vi "DataChunkingLabview.vi"() -> ()   [LabVIEW 2019]
uses:
  <vilib>/addons/database/NI_Database_API.lvlib
  MIs softarwer2/JSW BELLERA CODE/New gary MIS/Gary Coating Code MIS/Sub VIs/Thickness.llb/Thickness Global.vi
  <vilib>/addons/database/Connection.llb/DB Tools Open Connec (String).vi
  <vilib>/addons/database/Auxilliary.llb/DB Tools Parameter Dir.ctl
  <vilib>/addons/database/Auxilliary.llb/DB Tools DataTypes.ctl
  <vilib>/addons/database/Auxilliary.llb/DB Tools Parameter Info.ctl
  <vilib>/addons/database/Command.llb/Cmd Set Parameter Value (C).vi
  <vilib>/addons/database/Auxilliary.llb/DB Tools Format Datetime String (Time Stamp).vi
  <vilib>/addons/database/Command.llb/Cmd Execute.vi
  <vilib>/addons/database/Recordset.llb/Rec Fetch Recordset Data (CR).vi
  <vilib>/addons/database/Command.llb/Cmd Delete.vi
  <vilib>/addons/database/Recordset.llb/Rec Destroy - Command.vi
panel:
  out "size(s)":i32[](array[numeric])
  in  "offset for Data":dbl
  in  "?":dbl
  out "no of iteration":i32
  out "Array":variant[][][](array[variant])
  in  "From  Date":timestamp
  out "Tota records":variant[][](array[variant])
  out "no of records from db":i32
  in  "To Date":timestamp
  out "element":variant
  out "initialized array":variant[](array[variant])
  out "date string 3":string
  out "time string 2":string
  out "date string 4":string
  out "time string 3":string
types:
  T1 = typedef "NI_Database_API.lvlib/Conn ObjectReference.ctl" = refnum<k1>
  T2 = typedef "NI_Database_API.lvlib/DB Tools Parameter Info.ctl" = cluster{"parameter name":string, "type":T3, "direction":T4, "value":variant}
  T3 = typedef "NI_Database_API.lvlib/DB Tools DataTypes.ctl" = enum16{"String", "Long (I32)", "Single (SGL)", "Double (DBL)", "Date/Time", "Binary"}
  T4 = typedef "NI_Database_API.lvlib/DB Tools Parameter Dir.ctl" = enum32{"Input", "Output", "Input/Output", "Return Value"}
  T5 = typedef "NI_Database_API.lvlib/Cmd ObjectReference.ctl" = refnum<k1>
  T6 = typedef "NI_Database_API.lvlib/Cmd-Rec Object Reference.ctl" = refnum<k1>
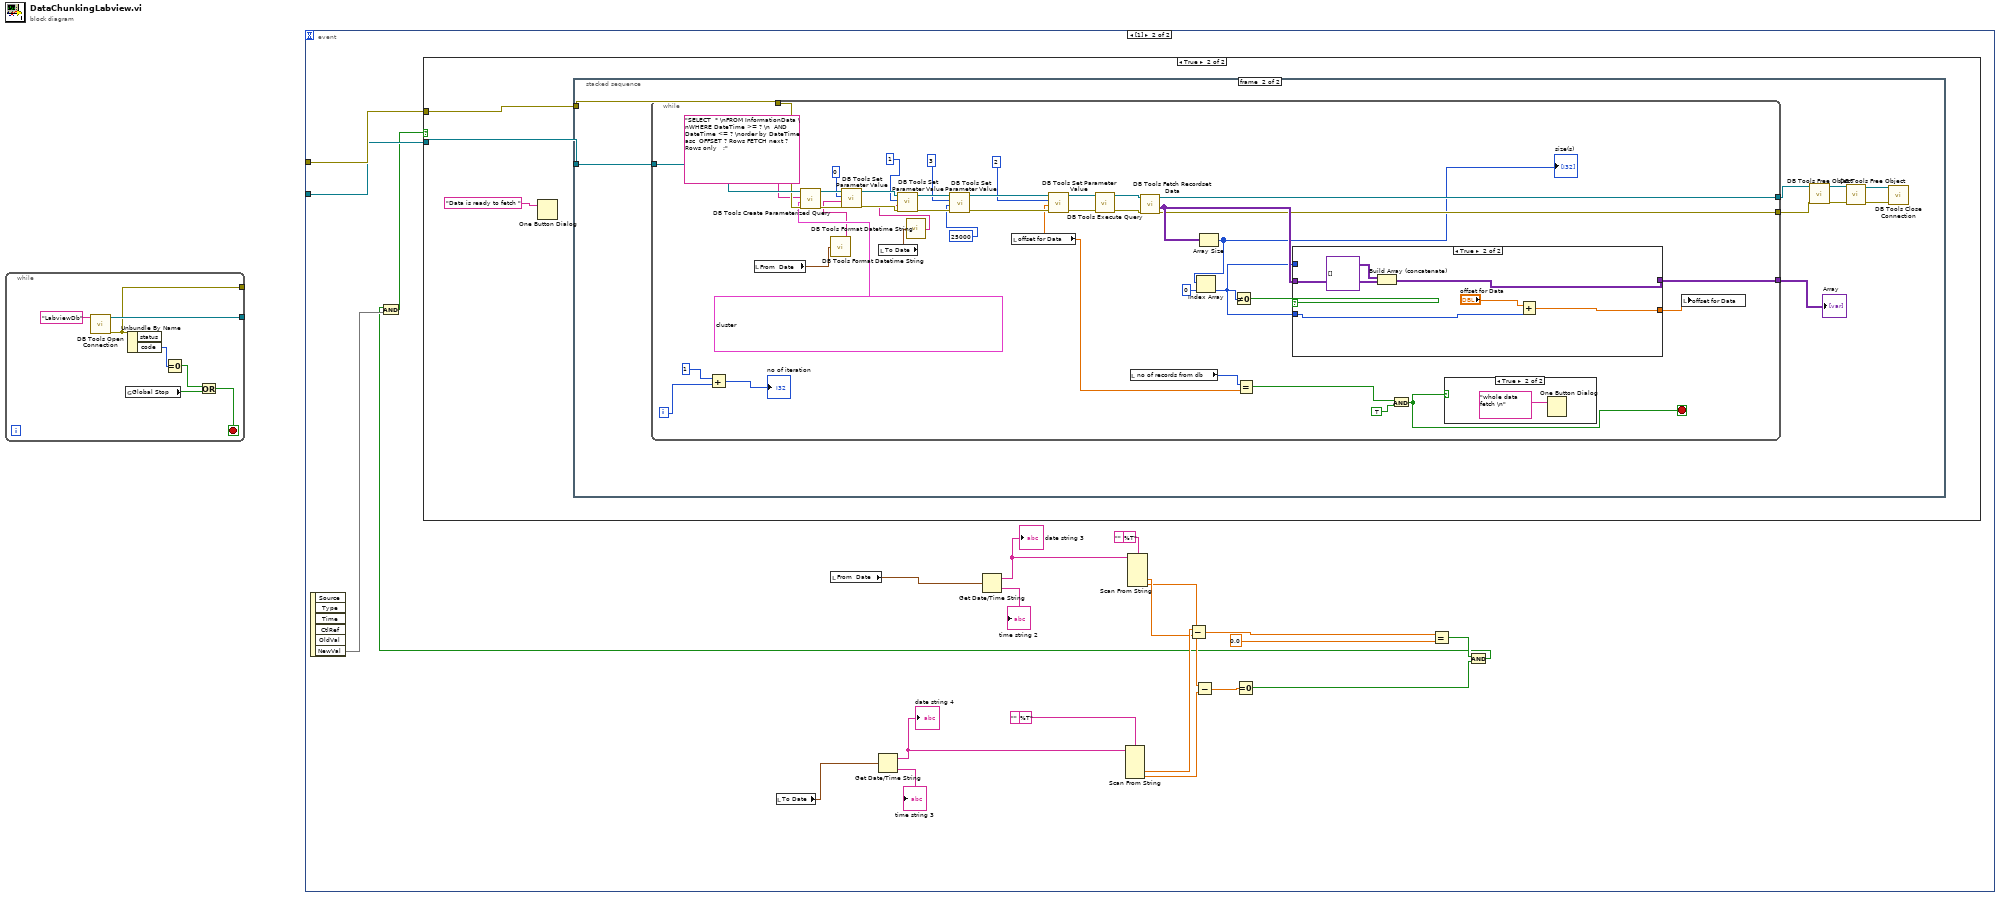
[diagram p0: block diagram]
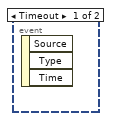
[diagram p2: hidden frame]
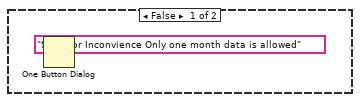
[diagram p3: hidden frame]
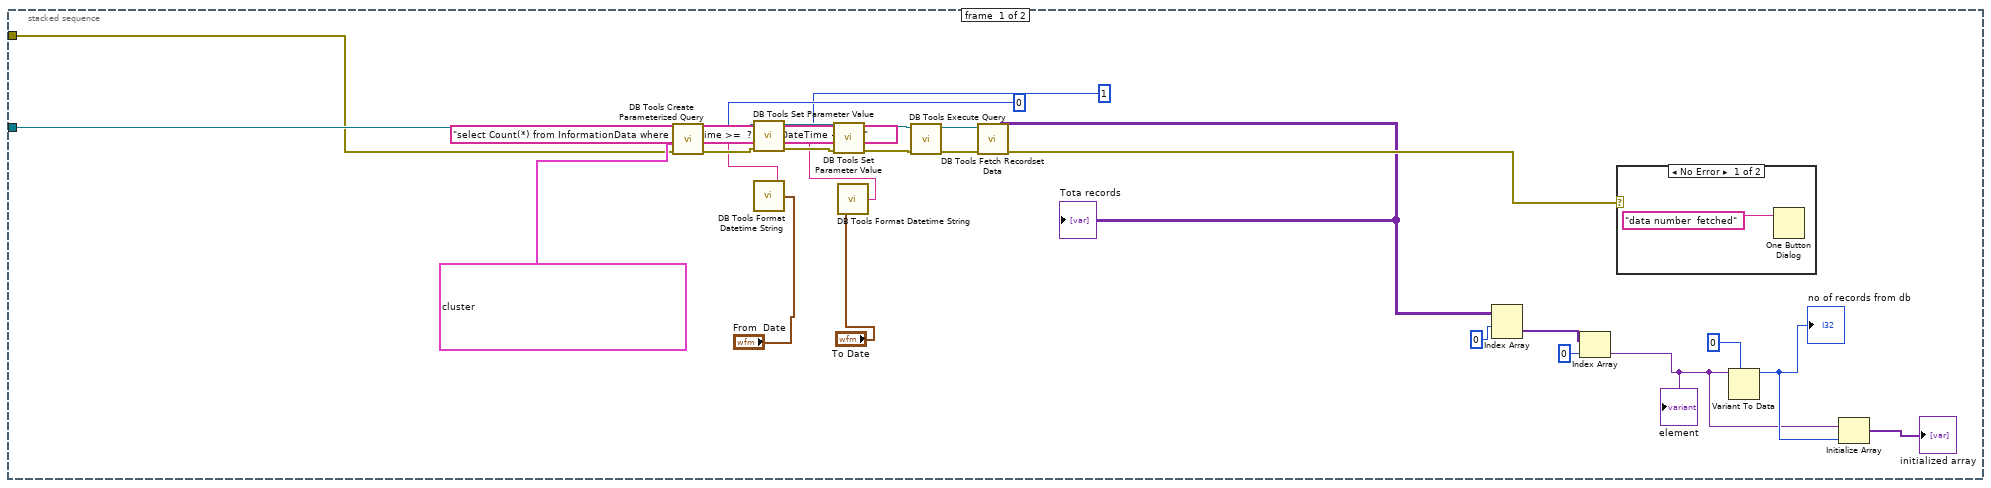
[diagram p4: hidden frame]
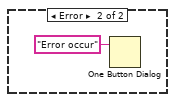
[diagram p5: hidden frame]
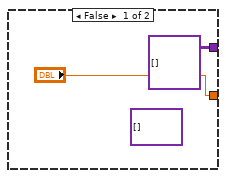
[diagram p7: hidden frame]
diagram:
  n1 = while {
    tunnel: [w2] -> _
    tunnel: [w1] -> _
    stop <- w3 stop-if-true
    n2 = call-poly <vilib>:"DB Tools Open Connection.vi"("connection information"="LabviewDb") -> ("error out"=w1:errorcluster, "connection reference"=w2:T1)  [unwired: 7 in]
    n3 = global read "Thickness Global.vi" "Global Stop"() -> (w4:bool)
    n4 = Unbundle By Name(w1) -> ("code"=w6:i32)  [unwired: 1 out]
    n5 = Equal To 0?(x=w6) -> (x = 0?=w5:bool)
    n6 = Or(x=w5, y=w4) -> (x .or. y?=w3:bool)
  }
  n7 = event shown="[1]" {
    selector: _ -> [_ _]
    dyn-events: _ -> [_ _]
    timeout: _ -> [_ _]
    tunnel: _ -> [_ w29]
    tunnel: _ -> [_ w28]
    event Timeout {
      n8 = event-data() -> ()  [unwired: 1 in, 3 out]
    }
    event #1 (no event record) {
      (unwired) "%T" ("format string")
      (unwired) "%T" ("format string")
      n9 = event-data() -> ("NewVal"=w27)  [unwired: 1 in, 5 out]
      n10 = local read "To Date"() -> (w8:timestamp)
      n11 = local read "From  Date"() -> (w9:timestamp)
      n12 = Get Date/Time String(seconds (now)=w8) -> (date string=w21:string, time string=→"time string 3":string)  [unwired: 2 in]
      "date string 4" <- w21
      n13 = Get Date/Time String(seconds (now)=w9) -> (date string=w24:string, time string=→"time string 2":string)  [unwired: 2 in]
      "date string 3" <- w24
      n14 = Scan From String(format string="", input string=w21) -> (output 2=w19:dbl, output 3=w14:dbl)  [unwired: 6 in, 3 out]
      n15 = Scan From String(format string="", input string=w24) -> (output 2=w18:dbl, output 3=w15:dbl)  [unwired: 6 in, 3 out]
      n16 = Subtract(x=w19, y=w18) -> (x-y=w16:dbl)
      n17 = Subtract(x=w15, y=w14) -> (x-y=w13:dbl)
      n18 = Equal To 0?(x=w13) -> (x = 0?=w11:bool)
      n19 = Equal?(x=w16, y=0.0) -> (x = y?=w12:bool)
      n20 = And(x=w12, y=w11) -> (x .and. y?=w10:bool)
      n21 = And(x=w10, y=w27) -> (x .and. y?=w26:bool)
      n22 = case shown="True" w26 {
        tunnel: w29 -> [_ w31]
        tunnel: w28 -> [_ w32]
        frame False {
          n23 = One Button Dialog(message="Sorry for Inconvience Only one month data is allowed") -> ()  [unwired: 1 in, 1 out]
        }
        frame True {
          n24 = One Button Dialog(message="Data is ready to fetch ") -> ()  [unwired: 1 in, 1 out]
          n25 = stacked-sequence {
            tunnel: w32 -> [w45 w71]
            tunnel: w31 -> [w44 w70]
            frame #0 {
              n26 = call <vilib>:"DB Tools Create Parameterized Query.vi"("error in (no error)"=w44, "parameters"=T2[] [{"parameter name"="fromDate", "type"=enum."Date/Time", "direction"=enum."Input", "value"=variant}, {"parameter name"="toDate", "type"=enum."Date/Time", "direction"=enum."Input", "value"=variant}], "SQL query"="select Count(*) from InformationData where  DateTime >=  ?  AND DateTime <= ?;  ", "connection reference"=w45) -> ("error out"=w57:errorcluster, "command reference"=w58:T5)  [unwired: 3 in, 1 out]
              n27 = call-poly <vilib>:"DB Tools Format Datetime String.vi"("time stamp"="From  Date") -> ("date/time string"=w55:string)
              n28 = call-poly <vilib>:"DB Tools Set Parameter Value.vi"("error in (no error)"=w57, "value"=w55, "parameter index"=0, "command reference"=w58) -> ("error out"=w53:errorcluster, "command reference out"=w54:T5)  [unwired: 4 in]
              n29 = call-poly <vilib>:"DB Tools Format Datetime String.vi"("time stamp"="To Date") -> ("date/time string"=w41:string)
              n30 = call-poly <vilib>:"DB Tools Set Parameter Value.vi"("error in (no error)"=w53, "value"=w41, "parameter index"=1, "command reference"=w54) -> ("error out"=w50:errorcluster, "command reference out"=w51:T5)  [unwired: 4 in]
              n31 = call-poly <vilib>:"DB Tools Execute Query.vi"("error in (no error)"=w50, "command reference"=w51) -> ("error out"=w48:errorcluster, "command-recordset reference"=w49:T6)  [unwired: 6 in]
              n32 = call-poly <vilib>:"DB Tools Fetch Recordset Data.vi"("error in (no error)"=w48, "command-recordset reference"=w49) -> ("error out"=w47:errorcluster, "recordset data"=w40:variant[][])  [unwired: 3 in, 1 out]
              "Tota records" <- w40
              n33 = Index Array(array=w40, index (row)=0 ("index")) -> (element=w39:variant[])  [unwired: 1 in]
              n34 = Index Array(array=w39, index=0) -> (element=w35:variant)
              "element" <- w35
              n35 = case shown="No Error" w47 {
                frame No Error {
                  n36 = One Button Dialog(message="data number  fetched") -> ()  [unwired: 1 in, 1 out]
                }
                frame Error {
                  n37 = One Button Dialog(message="Error occur") -> ()  [unwired: 1 in, 1 out]
                }
              }
              n38 = Variant To Data(type=0, Variant=w35) -> (data=w36:i32)  [unwired: 1 in, 1 out]
              "no of records from db" <- w36
              n39 = Initialize Array(w35, w36) -> (→"initialized array":variant[])
            }
            frame #1 {
              n40 = while {
                tunnel: w71 -> [w113]
                tunnel: w70 -> [w112]
                tunnel: [w77] -> w69
                tunnel: [w76] -> w68
                tunnel: [w72] -> w63
                i -> [w83]
                stop <- w73 stop-if-true
                n41 = Add(x=1, y=w83) -> (x+y=→"no of iteration":i32)
                n42 = local read "From  Date"() -> (w90:timestamp)
                n43 = call <vilib>:"DB Tools Create Parameterized Query.vi"("error in (no error)"=w112, "parameters"=T2[] [{"parameter name"="fromDate", "type"=enum."Date/Time", "direction"=enum."Input", "value"=variant}, {"parameter name"="toDate", "type"=enum."Date/Time", "direction"=enum."Input", "value"=variant}, {"parameter name"="fetch", "type"=enum."Long (I32)", "direction"=enum."Input", "value"=variant}, {"parameter name"="offset", "type"=enum."Long (I32)", "direction"=enum."Input", "value"=variant}], "SQL query"="SELECT  * \nFROM InformationData \nWHERE DateTime >= ? \n  AND DateTime <= ? \norder by DateTime asc  OFFSET ? Rows FETCH next ? Rows only   ;", "connection reference"=w113) -> ("error out"=w108:errorcluster, "command reference"=w109:T5)  [unwired: 3 in, 1 out]
                n44 = call-poly <vilib>:"DB Tools Format Datetime String.vi"("time stamp"=w90) -> ("date/time string"=w89:string)
                n45 = call-poly <vilib>:"DB Tools Set Parameter Value.vi"("error in (no error)"=w108, "value"=w89, "parameter index"=0, "command reference"=w109) -> ("error out"=w106:errorcluster, "command reference out"=w107:T5)  [unwired: 4 in]
                n46 = local read "To Date"() -> (w88:timestamp)
                n47 = call-poly <vilib>:"DB Tools Format Datetime String.vi"("time stamp"=w88) -> ("date/time string"=w87:string)
                n48 = call-poly <vilib>:"DB Tools Set Parameter Value.vi"("error in (no error)"=w106, "value"=w87, "parameter index"=1, "command reference"=w107) -> ("error out"=w104:errorcluster, "command reference out"=w105:T5)  [unwired: 4 in]
                n49 = call-poly <vilib>:"DB Tools Set Parameter Value.vi"("error in (no error)"=w104, "value"=25000, "parameter index"=3, "command reference"=w105) -> ("error out"=w102:errorcluster, "command reference out"=w103:T5)  [unwired: 4 in]
                n50 = local read "offset for Data"() -> (w78:dbl)
                n51 = call-poly <vilib>:"DB Tools Set Parameter Value.vi"("error in (no error)"=w102, "value"=w78, "parameter index"=2, "command reference"=w103) -> ("error out"=w96:errorcluster, "command reference out"=w95:T5)  [unwired: 4 in]
                n52 = call-poly <vilib>:"DB Tools Execute Query.vi"("error in (no error)"=w96, "command reference"=w95) -> ("error out"=w94:errorcluster, "command-recordset reference"=w93:T6)  [unwired: 6 in]
                n53 = local read "no of records from db"() -> (w91:i32)
                n54 = call-poly <vilib>:"DB Tools Fetch Recordset Data.vi"("error in (no error)"=w94, "command-recordset reference"=w93) -> ("error out"=w76:errorcluster, "recordset data"=w84:variant[][], "command-recordset reference out"=w77:T6)  [unwired: 3 in]
                n55 = Array Size(array=w84) -> (size(s)=w75:i32[])
                "size(s)" <- w75
                n56 = Index Array(array=w75, index=0 ("index (row)")) -> (element=w74:i32)
                n57 = Not Equal To 0?(x=w74) -> (x != 0?=w86:bool)
                n58 = Equal?(x=w91, y=w78) -> (x = y?=w80:bool)
                n59 = case shown="True" w86 {
                  tunnel: ["?" w121] -> w85
                  tunnel: w84 -> [_ w119]
                  tunnel: w74 -> [_ w120]
                  tunnel: w74 -> [_ _]
                  tunnel: [variant[][][] [] w117] -> w72
                  frame False {
                    (unwired) variant[][] [] ("array")
                  }
                  frame True {
                    n60 = Build Array (concatenate)(variant[][][] [] ("array"), w119) -> (w117:variant[][][])
                    n61 = Add(x="offset for Data", y=w120) -> (x+y=w121:dbl)
                  }
                }
                n62 = And(x=w80, y=TRUE) -> (x .and. y?=w73:bool)
                n63 = case shown="True" w73 {
                  frame False {
                  }
                  frame True {
                    n64 = One Button Dialog(message="whole data fetch \n") -> ()  [unwired: 1 in, 1 out]
                  }
                }
                n65 = local write "offset for Data"(w85) -> ()
              }
              "Array" <- w63
              n66 = call-poly <vilib>:"DB Tools Free Object.vi"("error in (no error)"=w68, "command-recordset reference"=w69) -> ("error out"=w67:errorcluster, "command reference"=w66:T5)  [unwired: 8 in]
              n67 = call-poly <vilib>:"DB Tools Free Object.vi"("error in (no error)"=w67, "command reference"=w66) -> ("error out"=w65:errorcluster, "connection reference"=w64:T1)  [unwired: 8 in]
              n68 = call <vilib>:"DB Tools Close Connection.vi"("error in (no error)"=w65, "connection reference"=w64) -> ()  [unwired: 5 in, 1 out]
            }
          }
        }
      }
    }
  }
